vi "_Destroy.vi"(8 "error in (no error)":errorcluster, 11 "Synapse CCD in":refnum<class "Synapse CCD.lvclass">) -> (0 "error out":errorcluster)   [LabVIEW 2012, in "Synapse CCD.lvclass"]
doc: "Superclass destructor: close all handles to and release all resources associated with this Instrument, then deallocate it. \n\nIMPORTANT: when destroying a class that inherits from Instrument, destroy your subclass first, and call the parent Instrument::_Destroy.vi LAST. This ensures your subclass destructor operates on a valid Instrument while it releases its resources."
uses:
  Synapse CCD.lvclass
  Utility Classes/Readable/Readable.lvclass
  Synapse CCD.lvclass/Synapse CCD.ctl
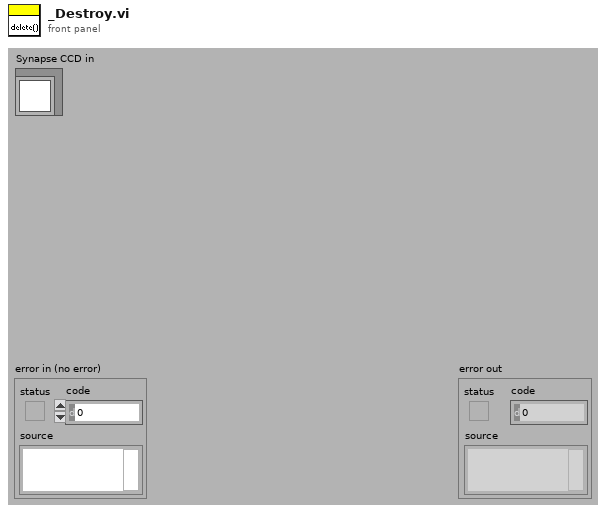
[diagram p1: front panel]
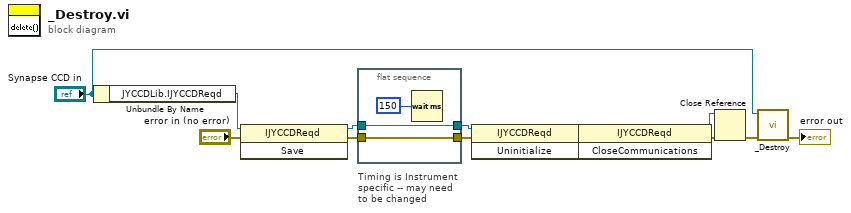
[diagram p0: block diagram]
diagram:
  n1 = Unbundle By Name("Synapse CCD in") -> ("JYCCDLib.IJYCCDReqd"=w11:refnum<k7>)
  n2 = invoke class="IJYCCDReqd" method="Save"(reference=w11, error in="error in (no error)") -> (reference out=w4:refnum<k7>, error out=w3:errorcluster)  [unwired: 1 in, 1 out]
  n3 = flat-sequence "Timing is Instrument\nspecific -- may need\nto be changed" {
    tunnel: w4 -> [w16]
    tunnel: w3 -> [w15]
    tunnel: [w16] -> w2
    tunnel: [w15] -> w1
    frame #0 {
      n4 = Wait (ms)(milliseconds to wait=u32 150) -> ()  [unwired: 1 out]
    }
  }
  n5 = invoke class="IJYCCDReqd" method="Uninitialize"(reference=w2, error in=w1) -> (reference out=w9:refnum<k7>, error out=w8:errorcluster)  [unwired: 1 in, 1 out]
  n6 = invoke class="IJYCCDReqd" method="CloseCommunications"(reference=w9, error in=w8) -> (reference out=w7:refnum<k7>, error out=w6:errorcluster)  [unwired: 1 in, 1 out]
  n7 = Close Reference(reference=w7, error in (no error)=w6) -> (error out=w5:errorcluster)
  n8 = call-parent "_Destroy.vi"("error in (no error)"=w5, "Instrument in"="Synapse CCD in") -> ("error out"=→"error out":errorcluster)  [unwired: 9 in]
